vi "Delay.vi"(6 "Button Mode":bool, 7 "Time Delay(s)":dbl, 9 "Elapsed Time Previous":dbl) -> (3 "Result":bool)   [LabVIEW 2018]
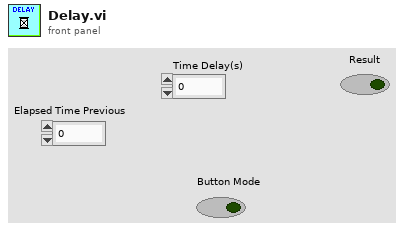
[diagram p1: front panel]
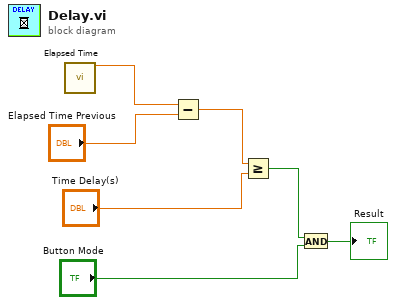
[diagram p0: block diagram]
diagram:
  n1 = call "Elapsed Time"() -> ("Present (s)"=w1:dbl)  [unwired: 12 in, 7 out]
  n2 = Subtract(x=w1, y="Elapsed Time Previous") -> (x-y=w6:dbl)
  n3 = Greater Or Equal?(x=w6, y="Time Delay(s)") -> (x >= y?=w3:bool)
  n4 = And(x=w3, y="Button Mode") -> (x .and. y?=→"Result":bool)
